vi "Send to Times.vi"(1 "max items per request":u8, 2 "#items":u16) -> (0 "for loop request":u16)   [LabVIEW 2014, in "Simatic S7.lvlib"]
uses:
  Simatic S7.lvlib
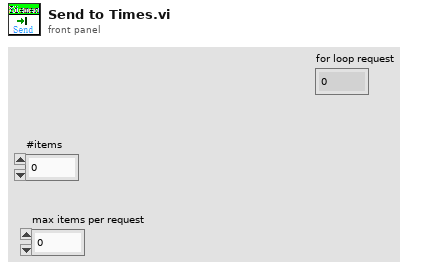
[diagram p1: front panel]
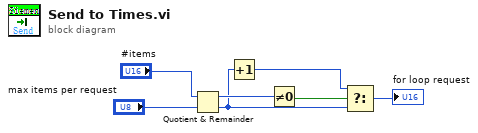
[diagram p0: block diagram]
diagram:
  n1 = Quotient & Remainder(x="#items", y="max items per request") -> (x-y*floor(x/y)=w5:u16, floor(x/y)=w3:u16)
  n2 = Increment(x=w3) -> (x+1=w2:u16)
  n3 = Not Equal To 0?(x=w5) -> (x != 0?=w4:bool)
  n4 = Select(t=w2, s=w4, f=w3) -> (s? t:f=→"for loop request":u16)
